vi "Get Caller Name.vi"() -> (0 "Name without Extension":string, 1 "Name with Extension":string)   [LabVIEW 2020, in "Utilities.lvlib"]
doc: "Gets the name of the caller of the VI's block diagram that this VI (Get Caller Name.vi) is placed on. The names are returned both with and without the file extension, which is typically \".vi\"."
uses:
  Utilities.lvlib
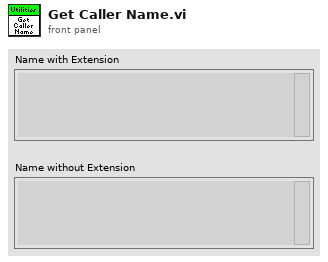
[diagram p1: front panel]
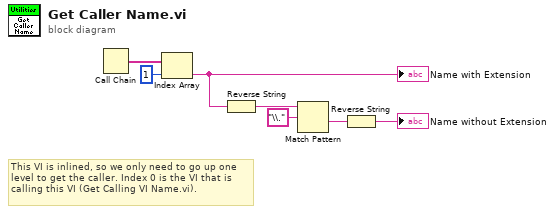
[diagram p0: block diagram]
diagram:
  # "This VI is inlined, so we only need to go up one level to get the caller. Index 0 is the VI that is calling this VI (Get Calling VI Name.vi)."
  n1 = Call Chain() -> (call chain=w7:string[])
  n2 = Index Array(array=w7, index=1) -> (element=w1:string)
  "Name with Extension" <- w1
  n3 = Reverse String(1:w1) -> (0:w5:string)
  n4 = Match Pattern(string=w5, regular expression="\\.") -> (after substring=w3:string)  [unwired: 1 in, 3 out]
  n5 = Reverse String(1:w3) -> (0:→"Name without Extension":string)
